vi "Set Tab Page.vi"(11 "Control Reference in":refnum<vi>) -> (0 "error out":errorcluster, 2 "Tab Control":enum32{"Display", "Settings"}(ring))   [LabVIEW 2016, in "Assert API Components.lvlib" / "Assert Display.lvlib" / "Main Display.lvlib" / "Main Display.lvclass"]
uses:
  Main Display.lvclass
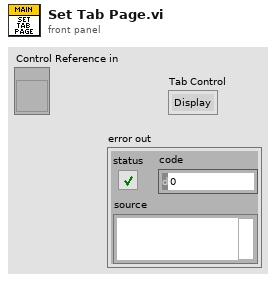
[diagram p1: front panel]
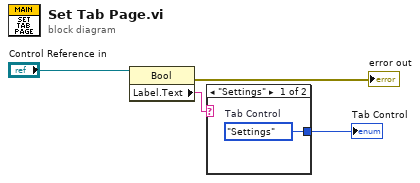
[diagram p0: block diagram]
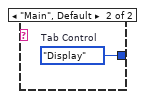
[diagram p2: hidden frame]
diagram:
  n1 = property class="Bool"(reference="Control Reference in") -> (error out=→"error out":errorcluster, "Label.Text"=w2:string)  [unwired: 1 in, 1 out]
  n2 = case shown="\"Settings\"" w2 {
    tunnel: [w5 w6] -> w3
    frame "Settings" {
      w5 = enum32{"Display", "Settings"}."Settings"  # Tab Control
    }
    frame "Main", Default {
      w6 = enum32{"Display", "Settings"}."Display"  # Tab Control
    }
  }
  "Tab Control" <- w3
